vi "refNewton Raphson Zero Finder numeric derivative.vi"(5 "function parameters":variant, 6 "accuracy":dbl=1e-08 format="%.2e", 7 "level":dbl, 8 "error in (no error)":errorcluster, 9 "end":dbl, 10 "start":dbl, 11 "function refnum":T1) -> (0 "error out":errorcluster, 2 "f(zero)":dbl format="%.2f", 3 "zero":dbl format="%.2f", 4 "f'(zero)":dbl)   [LabVIEW 2017, in "NI_Gmath.lvlib"]
doc: "Determines a zero of a 1D function close to two points with the help of the derivative of this 1D function. The two values form a search limit for the unknown zero of the 1D function."
uses:
  NI_Gmath.lvlib
  functionRefnum.ctl
panel:
  in  "function settings":T2
  in  "NR Settings":cluster{"accuracy":dbl, "max iterations":i32}={"accuracy"=1e-08, "max iterations"=200}
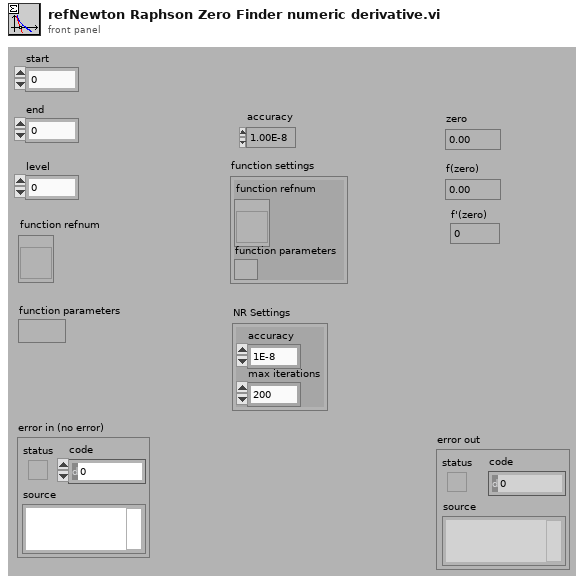
[diagram p1: front panel]
types:
  T1 = typedef "NI_Gmath.lvlib/functionRefnum.ctl" = refnum<vi>
  T2 = cluster{"function refnum":T1, "function parameters":variant}
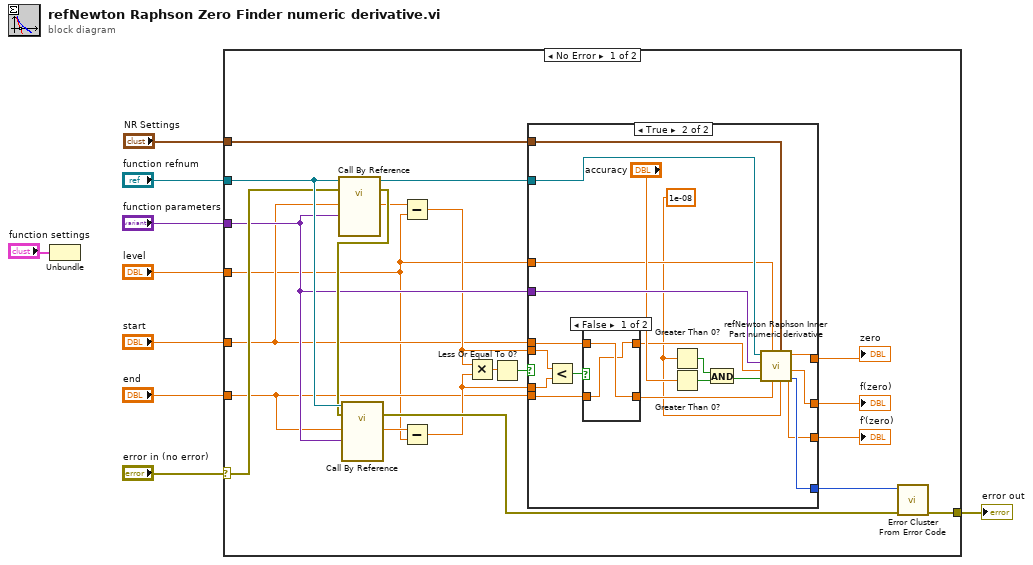
[diagram p0: block diagram]
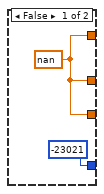
[diagram p2: hidden frame]
diagram:
  n1 = Unbundle("function settings") -> ()  [unwired: 2 out]
  n2 = case shown="No Error" "error in (no error)" {
    selector: "error in (no error)" -> [w27 w57]
    tunnel: "function refnum" -> [w28 _]
    tunnel: "function parameters" -> [w18 _]
    tunnel: [w24 w57] -> w6
    tunnel: "level" -> [w10 _]
    tunnel: "start" -> [w13 _]
    tunnel: "end" -> [w12 _]
    tunnel: "NR Settings" -> [w11 _]
    frame No Error {
      n3 = call-by-ref "?"(reference=w28, error in=w27, "Variant"=w18, "x"=w13) -> (reference out=w21:T1, error out=w20:errorcluster, "f(x)"=w17:dbl)  [unwired: 3 in]
      n4 = call-by-ref "?"(reference=w28, error in=w20, "Variant"=w18, "x"=w12) -> (error out=w19:errorcluster, "f(x)"=w15:dbl)  [unwired: 3 in, 1 out]
      n5 = Subtract(x=w17, y=w10) -> (x-y=w16:dbl)
      n6 = Subtract(x=w15, y=w10) -> (x-y=w14:dbl)
      n7 = Multiply(x=w16, y=w14) -> (x*y=w22:dbl)
      n8 = Less Or Equal To 0?(x=w22) -> (x <= 0?=w23:bool)
      n9 = case shown="True" w23 {
        tunnel: w13 -> [_ w42]
        tunnel: w12 -> [_ w41]
        tunnel: [w31 w35] -> w30
        tunnel: [w31 w34] -> w29
        tunnel: [-23021 w46] -> w25
        tunnel: w16 -> [_ w40]
        tunnel: w14 -> [_ w39]
        tunnel: w21 -> [_ w52]
        tunnel: w18 -> [_ w51]
        tunnel: [w31 w36] -> w26
        tunnel: w11 -> [_ w38]
        tunnel: w10 -> [_ w37]
        frame False {
          w31 = nan
        }
        frame True {
          w33 = 1e-08 ("h")
          n10 = Less?(x=w40, y=w39) -> (x < y?=w45:bool)
          n11 = case shown="False" w45 {
            tunnel: w42 -> [w54 w56]
            tunnel: w41 -> [w53 w55]
            tunnel: [w53 w56] -> w44
            tunnel: [w54 w55] -> w43
            frame False {
            }
            frame True {
            }
          }
          n12 = Greater Than 0?(x=w33) -> (x > 0?=w48:bool)
          n13 = Greater Than 0?(x="accuracy") -> (x > 0?=w49:bool)
          n14 = And(x=w48, y=w49) -> (x .and. y?=w47:bool)
          n15 = call "refNewton Raphson Inner Part numeric derivative.vi"("h"=w33, "NR Settings"=w38, "end/start"=w43, "level"=w37, "case"=w47, "start/end"=w44, "Variant"=w51, "function refnum"=w52) -> ("error"=w46:i32, "f(zero)"=w34:dbl, "f'(zero)"=w36:dbl, "zero"=w35:dbl)
        }
      }
      "zero" <- w30
      "f(zero)" <- w29
      "f'(zero)" <- w26
      n16 = call "Error Cluster From Error Code.vi"("error in (no error)"=w19, "error code (0)"=w25) -> ("error out"=w24:errorcluster)  [unwired: 1 in, 6 out]
    }
    frame Error {
    }
  }
  "error out" <- w6
